vi "Sub_VI_calculate.vi"(8 "Num 2":dbl, 9 "Combo Box":string(combo), 11 "Num 1":dbl) -> (0 "Result":dbl)   [LabVIEW 2016]
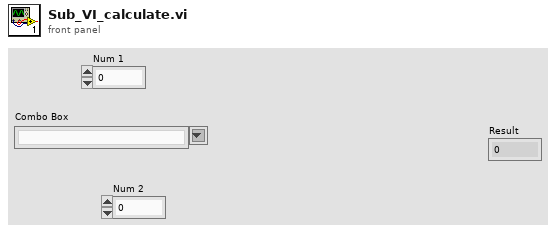
[diagram p1: front panel]
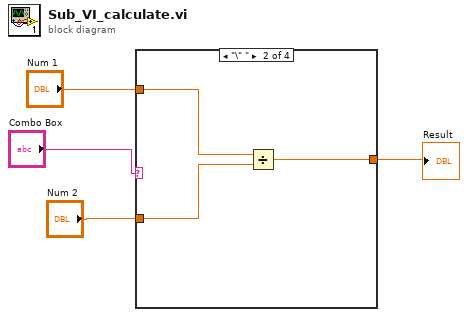
[diagram p0: block diagram]
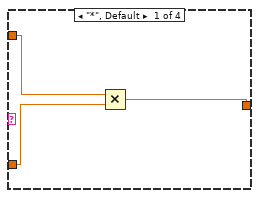
[diagram p2: hidden frame]
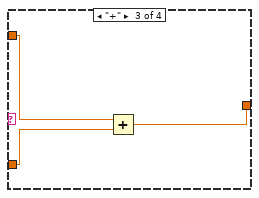
[diagram p3: hidden frame]
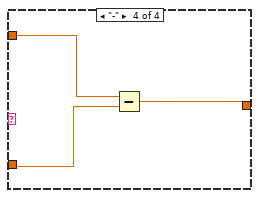
[diagram p4: hidden frame]
diagram:
  n1 = case shown="\"\\\" \"" "Combo Box" {
    tunnel: "Num 1" -> [w7 w10 w13 w16]
    tunnel: "Num 2" -> [w6 w9 w12 w15]
    tunnel: [w5 w8 w11 w14] -> w2
    frame "*", Default {
      n2 = Multiply(x=w7, y=w6) -> (x*y=w5:dbl)
    }
    frame "\" " {
      n3 = Divide(x=w10, y=w9) -> (x/y=w8:dbl)
    }
    frame "+" {
      n4 = Add(x=w13, y=w12) -> (x+y=w11:dbl)
    }
    frame "-" {
      n5 = Subtract(x=w16, y=w15) -> (x-y=w14:dbl)
    }
  }
  "Result" <- w2
